vi "multicolor creation 3(subvi).vi"(4 "on/off":bool[](array[boolean])=[TRUE, TRUE, TRUE], 5 "colors":T1(array[cluster]) {"min" step=0.01 format="%_2f"; "max" step=0.1 format="%_3f"}, 7 "fast/slow":bool, 9 "img array in":dbl[][][](array[numeric])=array1x90x160[14400 elements]) -> (1 "mixed img array":u32[][](array[numeric]), 2 "mixed img":picture)   [LabVIEW 2024]
panel:
  out "x-y 8":dbl
  out "x-y 7":dbl
  out "x-y 6":dbl
  out "x-y 4":dbl
  out "x-y 3":dbl
  out "x-y 2":dbl
  out "x-y":dbl
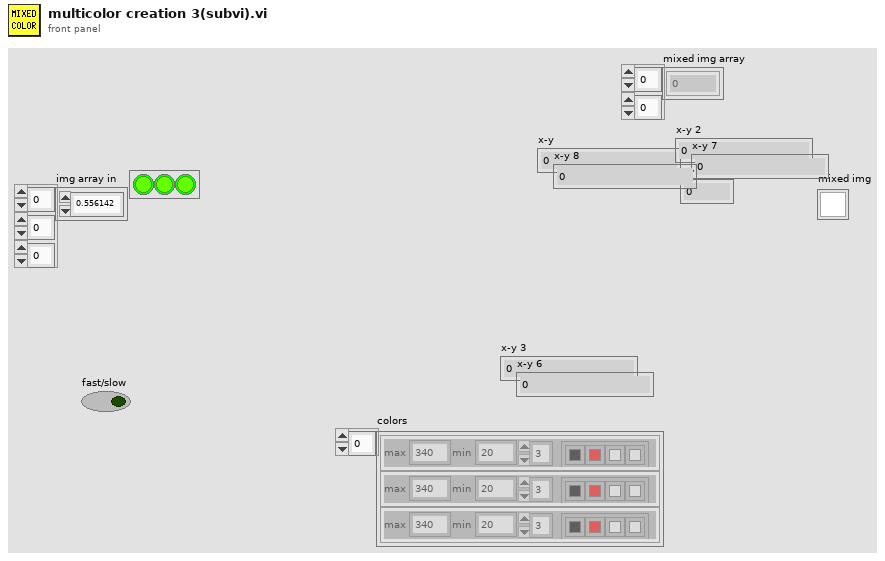
[diagram p1: front panel]
types:
  T1 = cluster{"color array":u32[], "num of colors":i32, "max":dbl, "min":dbl}[]
  T2 = typedef "imagedata.ctl" = cluster{"image type":i32, "image depth":i32, "image":u8[], "mask":u8[], "colors":u32[], "Rectangle":cluster{"left":i16, "top":i16, "right":i16, "bottom":i16}}
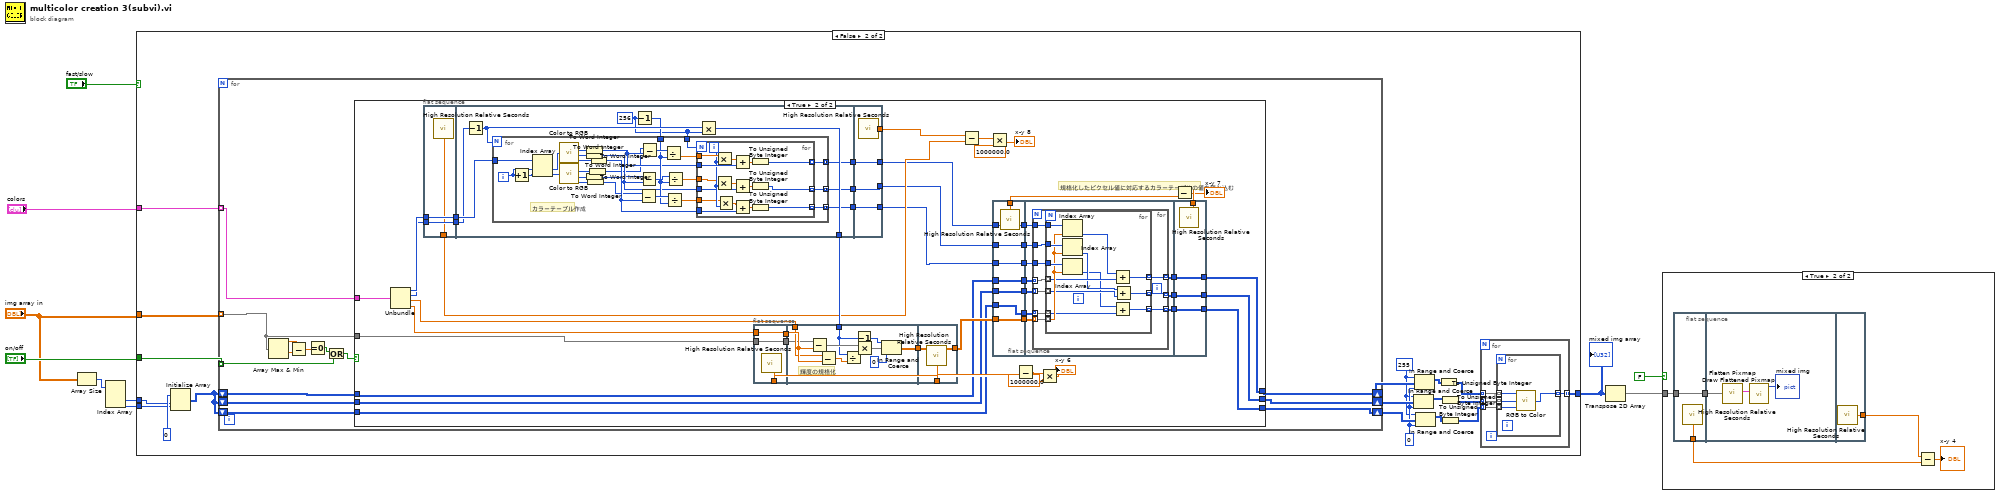
[diagram p0: block diagram]
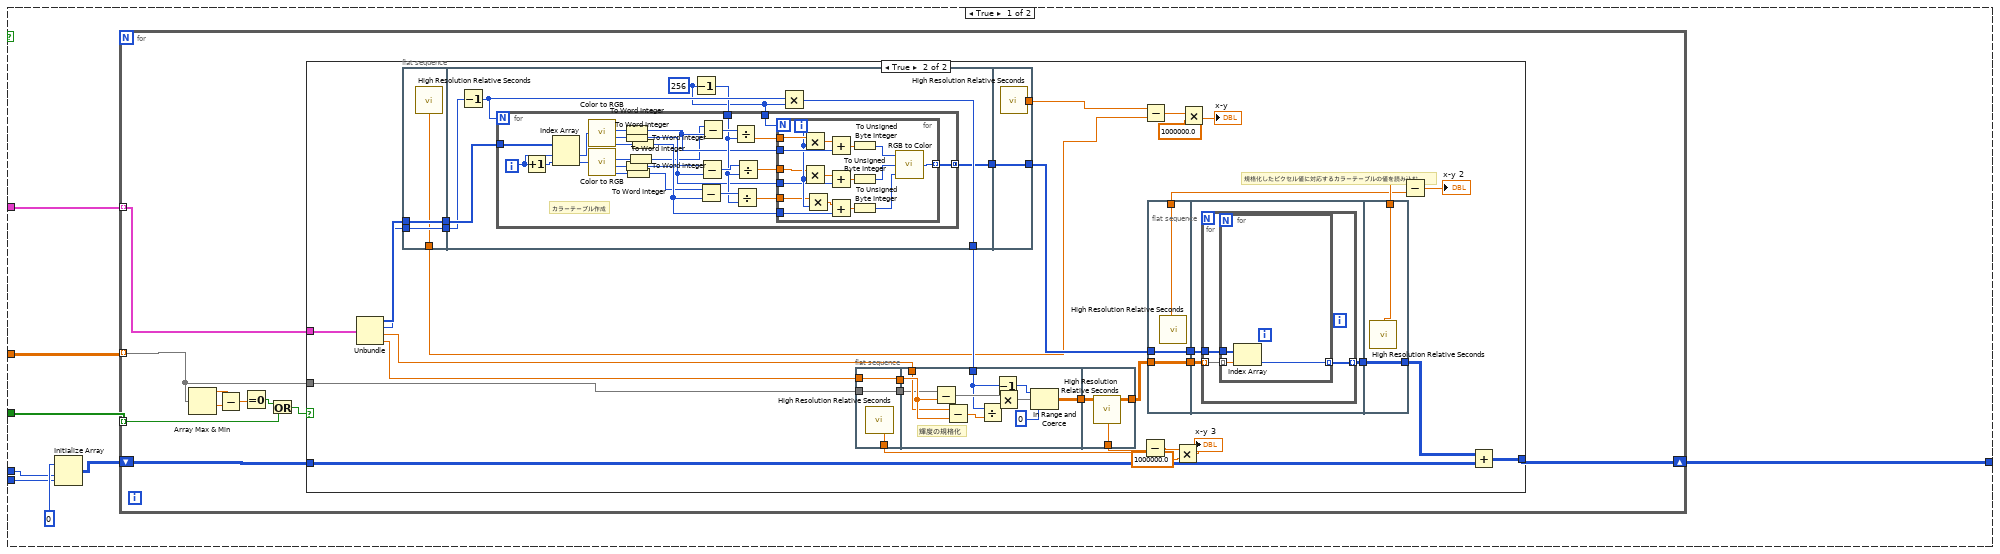
[diagram p3: hidden frame]
diagram:
  n1 = Array Size(array="img array in") -> (size(s)=w7:i32[])
  n2 = Index Array(array=w7) -> (element #2=w3:i32, element #3=w2:i32)  [unwired: 3 in, 1 out]
  n3 = case shown="False" "fast/slow" {
    tunnel: "colors" -> [w18 w167]
    tunnel: "on/off" -> [w17 w166]
    tunnel: "img array in" -> [w16 w165]
    tunnel: [w15 w149] -> w6
    tunnel: w3 -> [w13 w163]
    tunnel: w2 -> [w12 w162]
    frame True {
      n4 = Initialize Array(u32 0, w13, w12) -> (w11:u32[][])
      n5 = for {
        tunnel: w18 -> [w28] mode=indexing
        tunnel: w16 -> [w27] mode=indexing
        tunnel: w17 -> [w26] mode=indexing
        shift-right: [w25] -> w15
        shift-left: w11 -> [w24]
        n6 = Array Max & Min(array=w27) -> (max value=w23:dbl, min value=w22:dbl)  [unwired: 2 out]
        n7 = Subtract(x=w23, y=w22) -> (x-y=w21:dbl)
        n8 = Equal To 0?(x=w21) -> (x = 0?=w20:bool)
        n9 = Or(x=w20, y=w26) -> (x .or. y?=w19:bool)
        n10 = case shown="True" w19 {
          tunnel: w28 -> [_ w61]
          tunnel: w27 -> [_ w60]
          tunnel: [w29 w59] -> w25
          tunnel: w24 -> [w29 w58]
          frame False {
          }
          frame True {
            # "規格化したピクセル値に対応するカラーテーブルの値を読み込む"
            n11 = Unbundle(w61) -> ("color array"=w57:u32[], "num of colors"=w56:i32, "max"=w62:dbl, "min"=w63:dbl)
            n12 = flat-sequence {
              tunnel: w56 -> [w95]
              tunnel: w57 -> [w96]
              tunnel: [w96] -> w50
              tunnel: [w95] -> w49
              tunnel: [w94] -> w47
              tunnel: [w98] -> w55
              tunnel: [w97] -> w51
              tunnel: w50 -> [w103]
              tunnel: w49 -> [w102]
              tunnel: [w148] -> w54
              tunnel: w51 -> [w148]
              tunnel: [w147] -> w48
              frame #0 {
                n13 = call <vilib>:"High Resolution Relative Seconds.vi"() -> ("relative seconds"=w94:dbl)
              }
              frame #1 {
                w99 = u16 256 ("y")
                n14 = Decrement(x=w102) -> (x-1=w101:i32)
                n15 = Decrement(x=w99) -> (x-1=w100:u16)
                n16 = for {
                  N: w101 -> [_]
                  tunnel: w103 -> [w129]
                  tunnel: w100 -> [w116]
                  tunnel: w99 -> [w115]
                  tunnel: [w112] -> w97 mode=concatenating
                  i -> [w127]
                  # "カラーテーブル作成"
                  n17 = Increment(x=w127) -> (x+1=w128:i32)
                  n18 = Index Array(array=w129, index #1=w127, index #2=w128) -> (element #1=w126:u32, element #2=w125:u32)
                  n19 = call <vilib>:"Color to RGB.vi"("Color"=w126) -> ("R"=w123:u8, "G"=w111:u8, "B"=w110:u8)  [unwired: 1 out]
                  n20 = call <vilib>:"Color to RGB.vi"("Color"=w125) -> ("R"=w124:u8, "G"=w118:u8, "B"=w117:u8)  [unwired: 1 out]
                  n21 = To Word Integer(number=w123) -> (16bit integer=w109:i16)
                  n22 = To Word Integer(number=w111) -> (16bit integer=w108:i16)
                  n23 = To Word Integer(number=w118) -> (16bit integer=w105:i16)
                  n24 = To Word Integer(number=w117) -> (16bit integer=w104:i16)
                  n25 = To Word Integer(number=w124) -> (16bit integer=w106:i16)
                  n26 = To Word Integer(number=w110) -> (16bit integer=w107:i16)
                  n27 = Subtract(x=w104, y=w107) -> (x-y=w119:i16)
                  n28 = Subtract(x=w105, y=w108) -> (x-y=w120:i16)
                  n29 = Subtract(x=w106, y=w109) -> (x-y=w122:i16)
                  n30 = Divide(x=w122, y=w116) -> (x/y=w121:dbl)
                  n31 = Divide(x=w119, y=w116) -> (x/y=w113:dbl)
                  n32 = Divide(x=w120, y=w116) -> (x/y=w114:dbl)
                  n33 = for {
                    N: w115 -> [_]
                    tunnel: w109 -> [w145]
                    tunnel: w121 -> [w146]
                    tunnel: w114 -> [w137]
                    tunnel: w113 -> [w136]
                    tunnel: [w135] -> w112 mode=indexing
                    tunnel: w108 -> [w134]
                    tunnel: w107 -> [w133]
                    i -> [w138]
                    n34 = Multiply(x=w146, y=w138) -> (x*y=w141:dbl)
                    n35 = Multiply(x=w137, y=w138) -> (x*y=w142:dbl)
                    n36 = Multiply(x=w136, y=w138) -> (x*y=w139:dbl)
                    n37 = Add(x=w141, y=w145) -> (x+y=w144:dbl)
                    n38 = Add(x=w142, y=w134) -> (x+y=w143:dbl)
                    n39 = Add(x=w139, y=w133) -> (x+y=w140:dbl)
                    n40 = To Unsigned Byte Integer(number=w144) -> (unsigned 8bit integer=w132:u8)
                    n41 = To Unsigned Byte Integer(number=w143) -> (unsigned 8bit integer=w131:u8)
                    n42 = To Unsigned Byte Integer(number=w140) -> (unsigned 8bit integer=w130:u8)
                    n43 = call <vilib>:"RGB to Color.vi"("B"=w130, "G"=w131, "R"=w132) -> ("Color"=w135:u32)
                  }
                }
                n44 = Multiply(x=w101, y=w99) -> (x*y=w98:i32)
              }
              frame #2 {
                n45 = call <vilib>:"High Resolution Relative Seconds.vi"() -> ("relative seconds"=w147:dbl)
              }
            }
            n46 = flat-sequence {
              tunnel: w60 -> [w65]
              tunnel: w63 -> [w66]
              tunnel: [w66] -> w36
              tunnel: [w65] -> w35
              tunnel: [w64] -> w33
              tunnel: w62 -> [w76]
              tunnel: w55 -> [w69]
              tunnel: [w70] -> w37
              tunnel: w36 -> [w77]
              tunnel: w35 -> [w75]
              tunnel: [w79] -> w53
              tunnel: w37 -> [w79]
              tunnel: [w78] -> w34
              frame #0 {
                n47 = call <vilib>:"High Resolution Relative Seconds.vi"() -> ("relative seconds"=w64:dbl)
              }
              frame #1 {
                # "輝度の規格化"
                n48 = Subtract(x=w75, y=w77) -> (x-y=w72:dbl[][])
                n49 = Subtract(x=w76, y=w77) -> (x-y=w74:dbl)
                n50 = Divide(x=w69, y=w74) -> (x/y=w73:dbl)
                n51 = Decrement(x=w69) -> (x-1=w67:i32)
                n52 = Multiply(x=w72, y=w73) -> (x*y=w71:dbl[][])
                n53 = In Range and Coerce(upper limit=w67, x=w71, lower limit=0) -> (coerced(x)=w70:dbl[][])  [unwired: 1 out]
              }
              frame #2 {
                n54 = call <vilib>:"High Resolution Relative Seconds.vi"() -> ("relative seconds"=w78:dbl)
              }
            }
            n55 = Subtract(x=w34, y=w33) -> (x-y=w31:dbl)
            n56 = Subtract(x=w48, y=w47) -> (x-y=w46:dbl)
            n57 = flat-sequence {
              tunnel: w53 -> [w81]
              tunnel: w54 -> [w82]
              tunnel: [w82] -> w44
              tunnel: [w81] -> w43
              tunnel: [w80] -> w41
              tunnel: [w83] -> w45
              tunnel: w44 -> [w85]
              tunnel: w43 -> [w84]
              tunnel: [w93] -> w52
              tunnel: w45 -> [w93]
              tunnel: [w92] -> w42
              frame #0 {
                n58 = call <vilib>:"High Resolution Relative Seconds.vi"() -> ("relative seconds"=w80:dbl)
              }
              frame #1 {
                n59 = for {
                  tunnel: w85 -> [w88]
                  tunnel: w84 -> [w87] mode=indexing
                  tunnel: [w86] -> w83 mode=indexing
                  n60 = for {
                    tunnel: w88 -> [w91]
                    tunnel: w87 -> [w90] mode=indexing
                    tunnel: [w89] -> w86 mode=indexing
                    n61 = Index Array(array=w91, index=w90) -> (element=w89:u32)
                  }
                }
              }
              frame #2 {
                n62 = call <vilib>:"High Resolution Relative Seconds.vi"() -> ("relative seconds"=w92:dbl)
              }
            }
            n63 = Multiply(x=w31, y=1000000.0) -> (x*y=→"x-y 3":dbl)
            n64 = Multiply(x=w46, y=1000000.0) -> (x*y=→"x-y":dbl)
            n65 = Subtract(x=w42, y=w41) -> (x-y=→"x-y 2":dbl)
            n66 = Add(x=w52, y=w58) -> (x+y=w59:u32[][])
          }
        }
      }
    }
    frame False {
      w157 = 0
      w156 = 255
      n67 = Initialize Array(u16 0, w163, w162) -> (w161:u16[][])
      n68 = for {
        tunnel: w167 -> [w189] mode=indexing
        tunnel: w165 -> [w188] mode=indexing
        tunnel: w166 -> [w187] mode=indexing
        shift-right: [w186] -> w160
        shift-left: w161 -> [w185]
        shift-right: [w177] -> w159
        shift-left: w161 -> [w179]
        shift-right: [w176] -> w158
        shift-left: w161 -> [w178]
        n69 = Array Max & Min(array=w188) -> (max value=w184:dbl, min value=w183:dbl)  [unwired: 2 out]
        n70 = Subtract(x=w184, y=w183) -> (x-y=w182:dbl)
        n71 = Equal To 0?(x=w182) -> (x = 0?=w181:bool)
        n72 = Or(x=w181, y=w187) -> (x .or. y?=w180:bool)
        n73 = case shown="True" w180 {
          tunnel: w189 -> [_ w238]
          tunnel: w188 -> [_ w237]
          tunnel: [w192 w198] -> w186
          tunnel: w185 -> [w192 w203]
          tunnel: w179 -> [w191 w201]
          tunnel: w178 -> [w190 w199]
          tunnel: [w191 w196] -> w177
          tunnel: [w190 w194] -> w176
          frame False {
          }
          frame True {
            # "規格化したピクセル値に対応するカラーテーブルの値を読み込む"
            n74 = Unbundle(w238) -> ("color array"=w236:u32[], "num of colors"=w235:i32, "max"=w239:dbl, "min"=w240:dbl)
            n75 = flat-sequence {
              tunnel: w235 -> [w303]
              tunnel: w236 -> [w304]
              tunnel: [w304] -> w232
              tunnel: [w303] -> w231
              tunnel: [w302] -> w229
              tunnel: [w308] -> w234
              tunnel: w232 -> [w313]
              tunnel: w231 -> [w312]
              tunnel: [w307] -> w213
              tunnel: [w306] -> w212
              tunnel: [w305] -> w211
              tunnel: [w361] -> w230
              tunnel: [w360] -> w209
              tunnel: w213 -> [w360]
              tunnel: [w359] -> w207
              tunnel: w212 -> [w359]
              tunnel: [w358] -> w205
              tunnel: w211 -> [w358]
              frame #0 {
                n76 = call <vilib>:"High Resolution Relative Seconds.vi"() -> ("relative seconds"=w302:dbl)
              }
              frame #1 {
                w309 = u16 256 ("y")
                n77 = Decrement(x=w312) -> (x-1=w311:i32)
                n78 = Decrement(x=w309) -> (x-1=w310:u16)
                n79 = for {
                  N: w311 -> [_]
                  tunnel: w313 -> [w341]
                  tunnel: w310 -> [w328]
                  tunnel: w309 -> [w327]
                  tunnel: [w316] -> w307 mode=concatenating
                  tunnel: [w315] -> w306 mode=concatenating
                  tunnel: [w314] -> w305 mode=concatenating
                  i -> [w339]
                  # "カラーテーブル作成"
                  n80 = Increment(x=w339) -> (x+1=w340:i32)
                  n81 = Index Array(array=w341, index #1=w339, index #2=w340) -> (element #1=w338:u32, element #2=w337:u32)
                  n82 = call <vilib>:"Color to RGB.vi"("Color"=w338) -> ("R"=w335:u8, "G"=w324:u8, "B"=w323:u8)  [unwired: 1 out]
                  n83 = call <vilib>:"Color to RGB.vi"("Color"=w337) -> ("R"=w336:u8, "G"=w330:u8, "B"=w329:u8)  [unwired: 1 out]
                  n84 = To Word Integer(number=w335) -> (16bit integer=w322:i16)
                  n85 = To Word Integer(number=w324) -> (16bit integer=w321:i16)
                  n86 = To Word Integer(number=w330) -> (16bit integer=w318:i16)
                  n87 = To Word Integer(number=w329) -> (16bit integer=w317:i16)
                  n88 = To Word Integer(number=w336) -> (16bit integer=w319:i16)
                  n89 = To Word Integer(number=w323) -> (16bit integer=w320:i16)
                  n90 = Subtract(x=w317, y=w320) -> (x-y=w331:i16)
                  n91 = Subtract(x=w318, y=w321) -> (x-y=w332:i16)
                  n92 = Subtract(x=w319, y=w322) -> (x-y=w334:i16)
                  n93 = Divide(x=w334, y=w328) -> (x/y=w333:dbl)
                  n94 = Divide(x=w331, y=w328) -> (x/y=w325:dbl)
                  n95 = Divide(x=w332, y=w328) -> (x/y=w326:dbl)
                  n96 = for {
                    N: w327 -> [_]
                    tunnel: w322 -> [w356]
                    tunnel: w333 -> [w357]
                    tunnel: w326 -> [w348]
                    tunnel: w325 -> [w347]
                    tunnel: w321 -> [w346]
                    tunnel: w320 -> [w345]
                    tunnel: [w344] -> w316 mode=indexing
                    tunnel: [w343] -> w315 mode=indexing
                    tunnel: [w342] -> w314 mode=indexing
                    i -> [w349]
                    n97 = Multiply(x=w357, y=w349) -> (x*y=w352:dbl)
                    n98 = Multiply(x=w348, y=w349) -> (x*y=w353:dbl)
                    n99 = Multiply(x=w347, y=w349) -> (x*y=w350:dbl)
                    n100 = Add(x=w352, y=w356) -> (x+y=w355:dbl)
                    n101 = Add(x=w353, y=w346) -> (x+y=w354:dbl)
                    n102 = Add(x=w350, y=w345) -> (x+y=w351:dbl)
                    n103 = To Unsigned Byte Integer(number=w355) -> (unsigned 8bit integer=w344:u8)
                    n104 = To Unsigned Byte Integer(number=w354) -> (unsigned 8bit integer=w343:u8)
                    n105 = To Unsigned Byte Integer(number=w351) -> (unsigned 8bit integer=w342:u8)
                  }
                }
                n106 = Multiply(x=w311, y=w309) -> (x*y=w308:i32)
              }
              frame #2 {
                n107 = call <vilib>:"High Resolution Relative Seconds.vi"() -> ("relative seconds"=w361:dbl)
              }
            }
            n108 = flat-sequence {
              tunnel: w237 -> [w242]
              tunnel: w240 -> [w243]
              tunnel: [w243] -> w220
              tunnel: [w242] -> w219
              tunnel: [w241] -> w217
              tunnel: w239 -> [w253]
              tunnel: w234 -> [w246]
              tunnel: [w247] -> w221
              tunnel: w220 -> [w254]
              tunnel: w219 -> [w252]
              tunnel: [w256] -> w233
              tunnel: w221 -> [w256]
              tunnel: [w255] -> w218
              frame #0 {
                n109 = call <vilib>:"High Resolution Relative Seconds.vi"() -> ("relative seconds"=w241:dbl)
              }
              frame #1 {
                # "輝度の規格化"
                n110 = Subtract(x=w252, y=w254) -> (x-y=w249:dbl[][])
                n111 = Subtract(x=w253, y=w254) -> (x-y=w251:dbl)
                n112 = Divide(x=w246, y=w251) -> (x/y=w250:dbl)
                n113 = Decrement(x=w246) -> (x-1=w244:i32)
                n114 = Multiply(x=w249, y=w250) -> (x*y=w248:dbl[][])
                n115 = In Range and Coerce(upper limit=w244, x=w248, lower limit=0) -> (coerced(x)=w247:dbl[][])  [unwired: 1 out]
              }
              frame #2 {
                n116 = call <vilib>:"High Resolution Relative Seconds.vi"() -> ("relative seconds"=w255:dbl)
              }
            }
            n117 = Subtract(x=w230, y=w229) -> (x-y=w228:dbl)
            n118 = Multiply(x=w228, y=1000000.0) -> (x*y=→"x-y 8":dbl)
            n119 = flat-sequence {
              tunnel: w233 -> [w264]
              tunnel: [w264] -> w227
              tunnel: [w263] -> w225
              tunnel: [w262] -> w210
              tunnel: w209 -> [w262]
              tunnel: [w261] -> w208
              tunnel: w207 -> [w261]
              tunnel: [w260] -> w206
              tunnel: w205 -> [w260]
              tunnel: [w259] -> w204
              tunnel: w203 -> [w259]
              tunnel: [w258] -> w202
              tunnel: w201 -> [w258]
              tunnel: [w257] -> w200
              tunnel: w199 -> [w257]
              tunnel: w227 -> [w274]
              tunnel: w210 -> [w273]
              tunnel: w208 -> [w272]
              tunnel: w206 -> [w271]
              tunnel: w204 -> [w270]
              tunnel: w202 -> [w269]
              tunnel: w200 -> [w268]
              tunnel: [w267] -> w197
              tunnel: [w266] -> w195
              tunnel: [w265] -> w193
              tunnel: [w301] -> w226
              tunnel: [w300] -> w198
              tunnel: w197 -> [w300]
              tunnel: [w299] -> w196
              tunnel: w195 -> [w299]
              tunnel: [w298] -> w194
              tunnel: w193 -> [w298]
              frame #0 {
                n120 = call <vilib>:"High Resolution Relative Seconds.vi"() -> ("relative seconds"=w263:dbl)
              }
              frame #1 {
                n121 = for {
                  tunnel: w274 -> [w284] mode=indexing
                  tunnel: w273 -> [w283]
                  tunnel: w272 -> [w282]
                  tunnel: w271 -> [w281]
                  tunnel: w270 -> [w280] mode=indexing
                  tunnel: w269 -> [w279] mode=indexing
                  tunnel: w268 -> [w278] mode=indexing
                  tunnel: [w277] -> w267 mode=indexing
                  tunnel: [w276] -> w266 mode=indexing
                  tunnel: [w275] -> w265 mode=indexing
                  n122 = for {
                    tunnel: w284 -> [w294] mode=indexing
                    tunnel: w283 -> [w297]
                    tunnel: w282 -> [w296]
                    tunnel: w281 -> [w295]
                    tunnel: w280 -> [w293] mode=indexing
                    tunnel: w279 -> [w291] mode=indexing
                    tunnel: w278 -> [w289] mode=indexing
                    tunnel: [w287] -> w277 mode=indexing
                    tunnel: [w286] -> w276 mode=indexing
                    tunnel: [w285] -> w275 mode=indexing
                    n123 = Index Array(array=w297, index=w294) -> (element=w292:u8)
                    n124 = Index Array(array=w296, index=w294) -> (element=w290:u8)
                    n125 = Index Array(array=w295, index=w294) -> (element=w288:u8)
                    n126 = Add(x=w292, y=w293) -> (x+y=w287:u16)
                    n127 = Add(x=w288, y=w289) -> (x+y=w285:u16)
                    n128 = Add(x=w290, y=w291) -> (x+y=w286:u16)
                  }
                }
              }
              frame #2 {
                n129 = call <vilib>:"High Resolution Relative Seconds.vi"() -> ("relative seconds"=w301:dbl)
              }
            }
            n130 = Subtract(x=w218, y=w217) -> (x-y=w215:dbl)
            n131 = Multiply(x=w215, y=1000000.0) -> (x*y=→"x-y 6":dbl)
            n132 = Subtract(x=w226, y=w225) -> (x-y=→"x-y 7":dbl)
          }
        }
      }
      n133 = In Range and Coerce(upper limit=w156, x=w159, lower limit=w157) -> (coerced(x)=w154:i32[][])  [unwired: 1 out]
      n134 = In Range and Coerce(upper limit=w156, x=w160, lower limit=w157) -> (coerced(x)=w155:i32[][])  [unwired: 1 out]
      n135 = In Range and Coerce(upper limit=w156, x=w158, lower limit=w157) -> (coerced(x)=w153:i32[][])  [unwired: 1 out]
      n136 = To Unsigned Byte Integer(number=w155) -> (unsigned 8bit integer=w152:u8[][])
      n137 = To Unsigned Byte Integer(number=w154) -> (unsigned 8bit integer=w151:u8[][])
      n138 = To Unsigned Byte Integer(number=w153) -> (unsigned 8bit integer=w150:u8[][])
      n139 = for {
        tunnel: w152 -> [w171] mode=indexing
        tunnel: w151 -> [w170] mode=indexing
        tunnel: w150 -> [w169] mode=indexing
        tunnel: [w168] -> w149 mode=indexing
        n140 = for {
          tunnel: w171 -> [w175] mode=indexing
          tunnel: w170 -> [w174] mode=indexing
          tunnel: w169 -> [w173] mode=indexing
          tunnel: [w172] -> w168 mode=indexing
          n141 = call <vilib>:"RGB to Color.vi"("B"=w173, "G"=w174, "R"=w175) -> ("Color"=w172:u32)
        }
      }
    }
  }
  "mixed img array" <- w6
  n142 = Transpose 2D Array(2D array=w6) -> (transposed array=w5:u32[][])
  n143 = case shown="True" FALSE {
    tunnel: w5 -> [_ w365]
    frame False {
    }
    frame True {
      n144 = flat-sequence {
        tunnel: w365 -> [w368]
        tunnel: [w368] -> w366
        tunnel: [w367] -> w363
        tunnel: w366 -> [w369]
        tunnel: [w372] -> w364
        frame #0 {
          n145 = call <vilib>:"High Resolution Relative Seconds.vi"() -> ("relative seconds"=w367:dbl)
        }
        frame #1 {
          n146 = call <vilib>:"Flatten Pixmap.vi"("24-bit pixmap"=w369) -> ("image data"=w370:T2)  [unwired: 10 in]
          n147 = call <vilib>:"Draw Flattened Pixmap.vi"("image data"=w370) -> ("new picture"=→"mixed img":picture)  [unwired: 8 in]
        }
        frame #2 {
          n148 = call <vilib>:"High Resolution Relative Seconds.vi"() -> ("relative seconds"=w372:dbl)
        }
      }
      n149 = Subtract(x=w364, y=w363) -> (x-y=→"x-y 4":dbl)
    }
  }
